vi "Main.vi"(5 "Instructions":bool, 7 "Stop":T2, 8 "Path to saved file":path, 9 "Load Button":bool, 10 "Track Button":T1, 11 "Target Button":bool) -> (3 "String":string)   [LabVIEW 2018]
doc: "This VI displays the orientation of an Android smartphone."
uses:
  stop control.ctl
  track control 2.ctl
panel:
  out "y axis degrees":dbl(knob) caption="x axis degrees" scale=-180.0..180.0
  out "XY Graph":cluster{"X":dbl, "Y":dbl}[](graph)
  out "x axis degrees":dbl(knob) scale=-180.0..180.0
  out "In y axis":dbl
  out "In x axis":dbl
  in  "Instructions panel":enum32{"Page 1", "Page 2"}(tab)
  in  "DOT":bool=TRUE
  # "Orientation from targeted position"
  # "degrees"
  # "degrees"
  # "First make sure the mobile and the computer are in the same network!\n1) Open the app \"IMU+GPS-Stream\"\n2) Write the appropriate IP address of the machine running Labview\n3) Select \"UDP Stream\"\n4) Change panel to \"Toggle Sensors\" and select \"Orientation\" and \"Include User-Checked Sensor Data in Stream\"\n5) At the Preferences panel click \"Switch Stream\" and point the mobile to the screen\n6) After having the mobile face the screen, you can press the TARGET button to start seeing the orientation of your phone in accordance to the targeting you've made\n7) Alternatively:\n  - Press the TRACK button BEFORE pressing the TARGET button  to also enable the recording of the data.\n   - Press the LOAD button (after selecting an appropriate file) to load already existing data and view the recording"
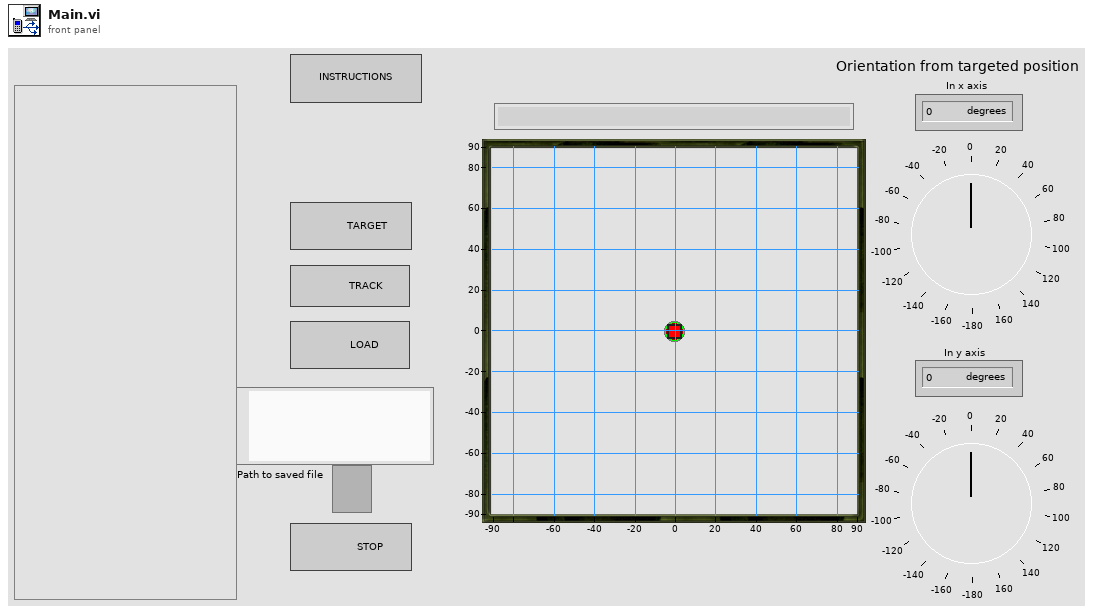
[diagram p1: front panel]
types:
  T1 = typedef "track control 2.ctl" = bool
  T2 = typedef "stop control.ctl" = bool
  T3 = enum16{"open", "replace", "create", "open or create", "replace or create", "replace or create with confirmation"}
  T4 = enum8{"Enabled", "Disabled", "Disabled and Grayed Out"}
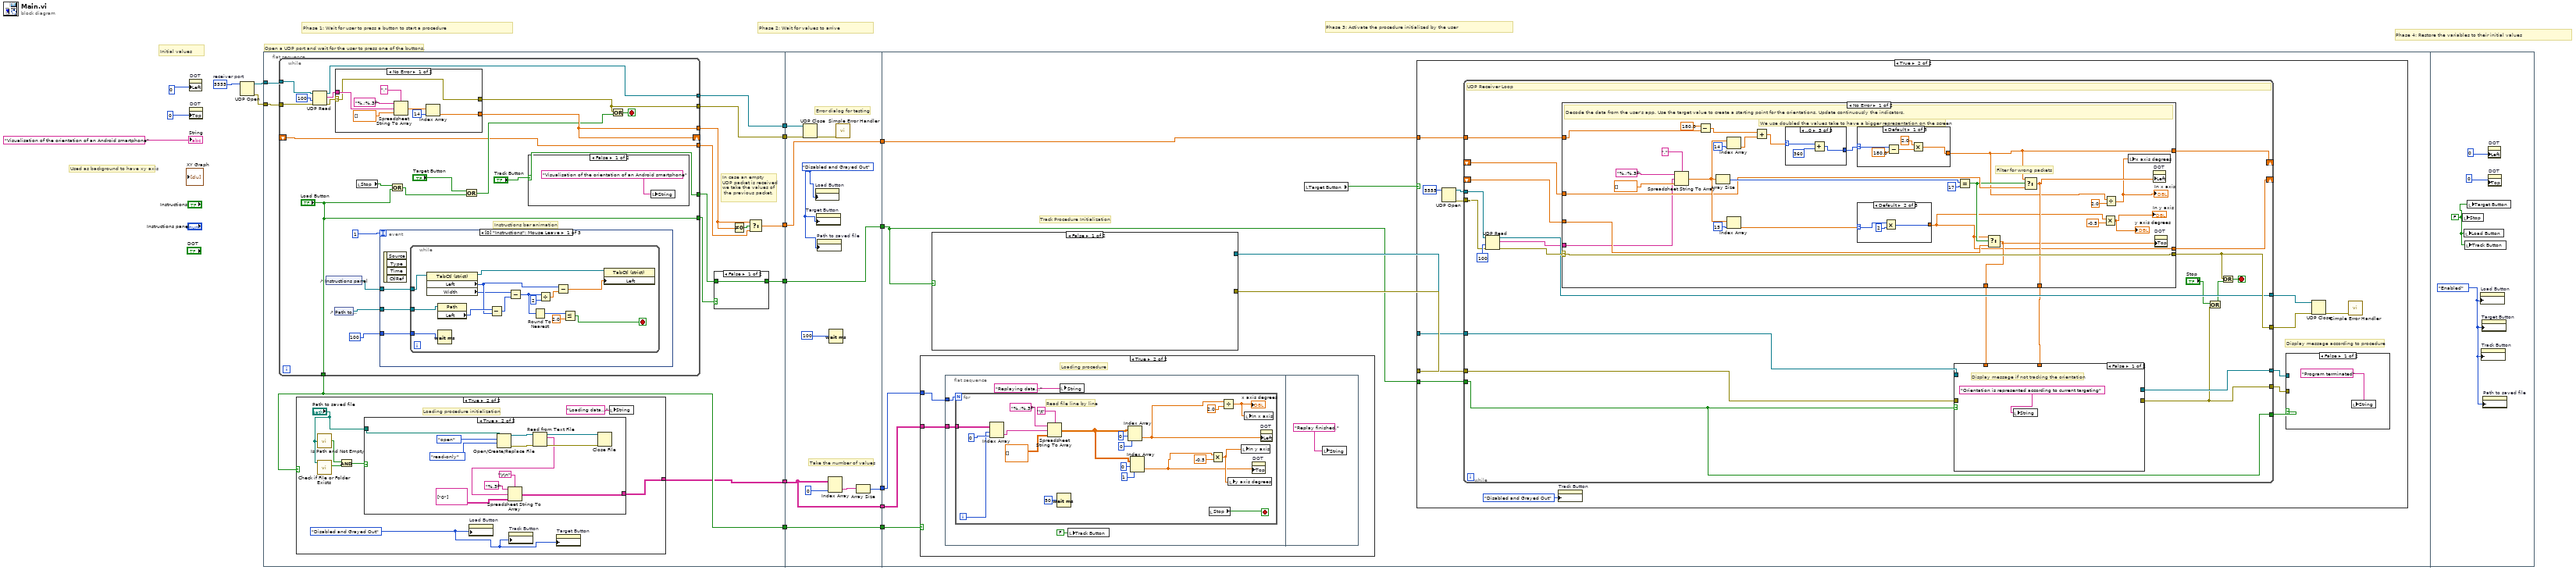
[diagram p0: block diagram]
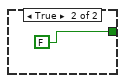
[diagram p2: hidden frame]
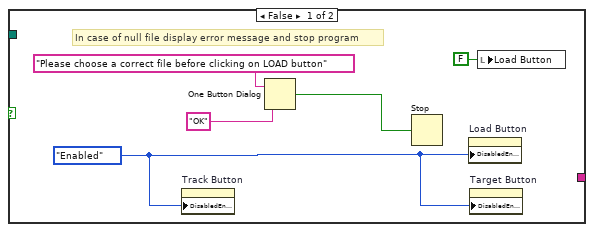
[diagram p4: hidden frame]
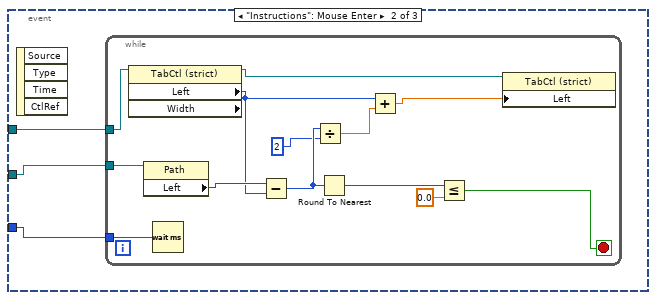
[diagram p5: hidden frame]
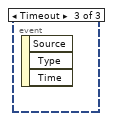
[diagram p6: hidden frame]
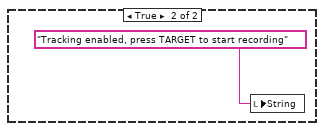
[diagram p7: hidden frame]
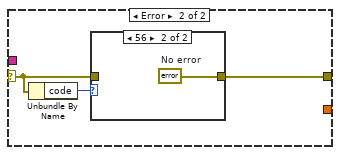
[diagram p8: hidden frame]
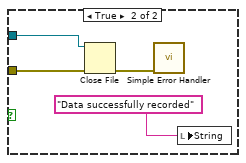
[diagram p11: hidden frame]
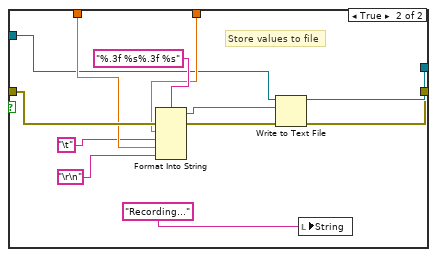
[diagram p12: hidden frame]
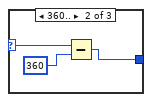
[diagram p14: hidden frame]
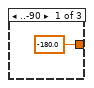
[diagram p15: hidden frame]
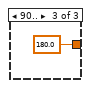
[diagram p16: hidden frame]
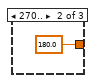
[diagram p17: hidden frame]
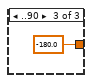
[diagram p18: hidden frame]
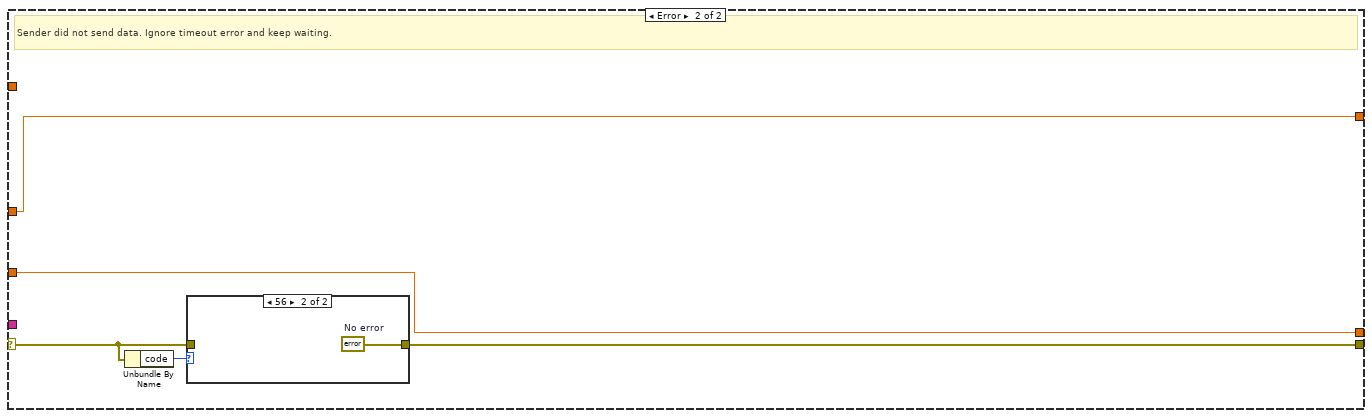
[diagram p19: hidden frame]
diagram:
  w17 = u16 5555  # receiver port
  # "Used as background to have xy axis"
  # "Phase 4: Restore the variables to their initial values"
  # "Phase 3: Activate the procedure initialized by the user"
  # "Phase 2: Wait for values to arrive"
  # "Phase 1: Wait for user to press a button to start a procedure"
  # "Open a UDP port and wait for the user to press one of the buttons."
  # "Initial values"
  n1 = property on="DOT" class="Bool (strict)"("Left"=0 ("Position:Left")) -> ()  [unwired: 2 in, 2 out]
  n2 = property on="DOT" class="Bool (strict)"("Top"=0 ("Position:Top")) -> ()  [unwired: 2 in, 2 out]
  n3 = UDP Open(11:w17) -> (port=w15:refnum<k16>, 0:w16:errorcluster)  [unwired: 4 in, 1 out]
  n4 = flat-sequence {
    tunnel: w15 -> [w28]
    tunnel: w16 -> [w27]
    tunnel: [w30] -> w14
    tunnel: [w29] -> w13
    tunnel: [w25] -> w12
    tunnel: [w22] -> w7
    tunnel: [w21] -> w5
    tunnel: [w18] -> w1
    tunnel: w14 -> [w135]
    tunnel: w13 -> [w136]
    tunnel: w12 -> [w134]
    tunnel: [w134] -> w11
    tunnel: [w133] -> w8
    tunnel: w7 -> [w133]
    tunnel: [w131] -> w6
    tunnel: w5 -> [w131]
    tunnel: [w129] -> w4
    tunnel: [w127] -> w2
    tunnel: w1 -> [w127]
    tunnel: w11 -> [w145]
    tunnel: w8 -> [w143]
    tunnel: w6 -> [w141]
    tunnel: w4 -> [w138]
    tunnel: w2 -> [w139]
    frame #0 {
      # "In case an empty\nUDP packet is received\nwe take the values of\n the previous packet."
      n5 = while {
        tunnel: w28 -> [w74]
        tunnel: [w72] -> w30
        tunnel: w27 -> [w75]
        tunnel: [w70] -> w29
        tunnel: [w69] -> w24
        shift-right: [w69] -> _
        shift-left: _ -> [w57]
        tunnel: [w57] -> w23
        tunnel: ["Load Button"] -> w22
        tunnel: ["Track Button"] -> w19
        tunnel: ["Load Button"] -> w20
        stop <- w62 stop-if-true
        # "Instructions bar animation"
        n6 = UDP Read(connection ID=w74, timeout ms (25000)=100, 8:w75) -> (data out=w73:string, error out=w71:errorcluster, 3:w72:refnum<k16>)  [unwired: 3 out]
        n7 = control-ref of="Instructions panel"() -> (w60:refnum<vi>)
        n8 = control-ref of="Path to saved file"() -> (w61:refnum<vi>)
        n9 = case shown="No Error" w71 {
          selector: w71 -> [w114 w122]
          tunnel: w73 -> [w116 _]
          tunnel: [w114 w121] -> w70
          tunnel: [w113 _] -> w69
          frame No Error {
            n10 = Spreadsheet String To Array(delimiter (Tab)=",", format string="%.;%.3f", spreadsheet string=w116, array type (2D Dbl)=dbl[] []) -> (array=w115:dbl[])
            n11 = Index Array(array=w115, index=14) -> (element=w113:dbl)
          }
          frame Error {
            n12 = Unbundle By Name(w122) -> ("code"=w123:i32)
            n13 = case shown="56" w123 {
              tunnel: w122 -> [w124 _]
              tunnel: [w124 w125] -> w121
              frame Default {
              }
              frame 56 {
                w125 = errorcluster {"status"=FALSE, "code"=0, "source"=""}  # No error
              }
            }
          }
        }
        n14 = local read "Stop"() -> (w66:T2)
        n15 = event shown="[0] \"Instructions\": Mouse Leave" {
          selector: _ -> [_ _ _]
          dyn-events: _ -> [_ _ _]
          timeout: 1 -> [_ _ _]
          tunnel: w61 -> [w79 w96 _]
          tunnel: w60 -> [w78 w95 _]
          tunnel: u32 100 ("Delay") -> [w77 w97 _]
          event "Instructions": Mouse Leave {
            n16 = event-data() -> ()  [unwired: 1 in, 4 out]
            n17 = while {
              tunnel: w79 -> [w91]
              tunnel: w78 -> [w90]
              tunnel: w77 -> [w89]
              stop <- w80 stop-if-true
              n18 = property on="Property Node" class="TabCtl (strict)"(reference=w90) -> (reference out=w92:refnum<vi>, "Left"=w93:i32, "Width"=w84:u32)  [unwired: 1 in, 1 out]
              n19 = property on="Property Node" class="Path"(reference=w91) -> ("Left"=w94:i32)  [unwired: 1 in, 2 out]
              n20 = Wait (ms)(milliseconds to wait=w89) -> ()  [unwired: 1 out]
              n21 = Subtract(x=w94, y=w93) -> (x-y=w87:i32)
              n22 = Subtract(x=w84, y=w87) -> (x-y=w88:u32)
              n23 = Round To Nearest(number=w88) -> (nearest integer value=w86:u32)
              n24 = Divide(x=w88, y=2) -> (x/y=w85:dbl)
              n25 = Subtract(x=w93, y=w85) -> (x-y=w81:dbl)
              n26 = Less Or Equal?(x=w86, y=2.0) -> (x <= y?=w80:bool)
              n27 = property on="Property Node" class="TabCtl (strict)"(reference=w92, "Left"=w81) -> ()  [unwired: 1 in, 2 out]
            }
          }
          event "Instructions": Mouse Enter {
            n28 = event-data() -> ()  [unwired: 1 in, 4 out]
            n29 = while {
              tunnel: w97 -> [w100]
              tunnel: w96 -> [w99]
              tunnel: w95 -> [w98]
              stop <- w101 stop-if-true
              n30 = property on="Property Node" class="TabCtl (strict)" props=["Left", "Width"](reference=w98) -> (reference out=w104:refnum<vi>, "Left"=w105:i32)  [unwired: 1 in, 2 out]
              n31 = property on="Property Node" class="Path"(reference=w99) -> ("Left"=w106:i32)  [unwired: 1 in, 2 out]
              n32 = Wait (ms)(milliseconds to wait=w100) -> ()  [unwired: 1 out]
              n33 = Subtract(x=w106, y=w105) -> (x-y=w107:i32)
              n34 = Divide(x=w107, y=2) -> (x/y=w109:dbl)
              n35 = Round To Nearest(number=w107) -> (nearest integer value=w108:i32)
              n36 = Add(x=w105, y=w109) -> (x+y=w110:dbl)
              n37 = Less Or Equal?(x=w108, y=0.0) -> (x <= y?=w101:bool)
              n38 = property on="Property Node" class="TabCtl (strict)"(reference=w104, "Left"=w110) -> ()  [unwired: 1 in, 2 out]
            }
          }
          event Timeout {
            n39 = event-data() -> ()  [unwired: 1 in, 3 out]
          }
        }
        n40 = Or(x=w66, y="Load Button") -> (x .or. y?=w65:T2)
        n41 = Or(x="Target Button", y=w65) -> (x .or. y?=w67:T2)
        n42 = case shown="False" "Track Button" {
          frame False {
            n43 = local write "String"("Visualisation of the orientation of an Android smartphone" ("String")) -> ()
          }
          frame True {
            n44 = local write "String"("Tracking enabled, press TARGET to start recording" ("String")) -> ()
          }
        }
        n45 = Or(x=w70, y=w67) -> (x .or. y?=w62:T2)
      }
      n46 = case shown="True" w22 {
        tunnel: [_ w39] -> w21
        frame False {
        }
        frame True {
          w33 = T4."Disabled and Grayed Out" ("Disabled")
          # "Loading procedure initialization"
          n47 = call <vilib>:"Is Path and Not Empty.vi"("path"="Path to saved file") -> ("Is Path and Not Empty?"=w36:bool)  [unwired: 4 in]
          n48 = call <vilib>:"Check if File or Folder Exists.vi"("path"="Path to saved file") -> ("file or folder exists?"=w37:bool)  [unwired: 8 in, 2 out]
          n49 = And(x=w36, y=w37) -> (x .and. y?=w35:bool)
          n50 = case shown="True" w35 {
            tunnel: [_ w46] -> w39
            tunnel: "Path to saved file" -> [_ w45]
            frame False {
              w41 = T4."Enabled" ("Disabled")
              # "In case of null file display error message and stop program"
              n51 = property on="Track Button" class="Bool (strict)"("DisabledEnum"=w41) -> ()  [unwired: 2 in, 2 out]
              n52 = One Button Dialog(message="Please choose a correct file before clicking on LOAD button", button name ("OK")="OK") -> (true=w42:bool)
              n53 = Stop(stop? (T)=w42) -> ()
              n54 = property on="Load Button" class="Bool (strict)"("DisabledEnum"=w41) -> ()  [unwired: 2 in, 2 out]
              n55 = property on="Target Button" class="Bool (strict)"("DisabledEnum"=w41) -> ()  [unwired: 2 in, 2 out]
              n56 = local write "Load Button"(FALSE ("Load Button")) -> ()
            }
            frame True {
              n57 = Open/Create/Replace File(file path (use dialog)=w45, operation (0:open)=T3."open", access (0:read/write)=enum16{"read/write", "read-only", "write-only"}."read-only") -> (refnum out=w51:refnum<file>, error out=w52:errorcluster)  [unwired: 3 in, 1 out]
              n58 = Read from Text File(file (use dialog)=w51, error in=w52) -> (refnum out=w56:refnum<file>, text=w50:string, error out=w55:errorcluster)  [unwired: 2 in, 1 out]
              n59 = Spreadsheet String To Array(delimiter (Tab)="\r\n", format string="%.3f", spreadsheet string=w50, array type (2D Dbl)=string[][] [["0"]]) -> (array=w46:string[][])
              n60 = Close File(refnum=w56, error in=w55) -> ()  [unwired: 2 out]
            }
          }
          n61 = property on="Load Button" class="Bool (strict)"("DisabledEnum"=w33) -> ()  [unwired: 2 in, 2 out]
          n62 = property on="Track Button" class="Bool (strict)"("DisabledEnum"=w33) -> ()  [unwired: 2 in, 2 out]
          n63 = property on="Target Button" class="Bool (strict)"("DisabledEnum"=w33) -> ()  [unwired: 2 in, 2 out]
          n64 = local write "String"("Loading data..." ("String")) -> ()
        }
      }
      n65 = case shown="False" w20 {
        tunnel: w19 -> [w31 _]
        tunnel: [w31 FALSE ("Track Button")] -> w18
        frame False {
        }
        frame True {
        }
      }
      n66 = Not Equal To 0?(x=w24) -> (x != 0?=w26:bool)
      n67 = Select(t=w24, s=w26, f=w23) -> (s? t:f=w25:dbl)
    }
    frame #1 {
      w126 = T4."Disabled and Grayed Out" ("Disabled")
      # "Error dialog for testing"
      # "Take the number of values"
      n68 = UDP Close(connection ID=w135, 8:w136) -> (error out=w128:errorcluster)  [unwired: 1 out]
      n69 = property on="Load Button" class="Bool (strict)"("DisabledEnum"=w126) -> ()  [unwired: 2 in, 2 out]
      n70 = property on="Target Button" class="Bool (strict)"("DisabledEnum"=w126) -> ()  [unwired: 2 in, 2 out]
      n71 = property on="Path to saved file" class="Path"("DisabledEnum"=w126) -> ()  [unwired: 2 in, 2 out]
      n72 = Index Array "Index Array"(array=w131, index (col)=0 ("index (row)")) -> (element=w130:string[])  [unwired: 1 in]
      n73 = Wait (ms)(milliseconds to wait=u32 100) -> ()  [unwired: 1 out]
      n74 = call <vilib>:"Simple Error Handler.vi"("error in (no error)"=w128) -> ()  [unwired: 1 in, 8 out]
      n75 = Array Size(array=w130) -> (size(s)=w129:i32)
    }
    frame #2 {
      # "Track Procedure Initialization"
      n76 = case shown="True" w143 {
        tunnel: w141 -> [_ w255]
        tunnel: w138 -> [_ w254]
        frame False {
        }
        frame True {
          # "Loading procedure"
          n77 = flat-sequence {
            tunnel: w255 -> [w259]
            tunnel: w254 -> [w258]
            frame #0 {
              n78 = for {
                N: w258 -> [_]
                tunnel: w259 -> [w279]
                i -> [w273]
                stop <- w266 stop-if-true
                # "Read file line by line"
                n79 = Index Array(array=w279, index (row)=w273, index (col)=0 ("index (row)")) -> (element=w278:string)
                n80 = Spreadsheet String To Array(delimiter (Tab)="\t", format string="%.;%.3f", spreadsheet string=w278, array type (2D Dbl)=dbl[][] []) -> (array=w268:dbl[][])
                n81 = Wait (ms)(milliseconds to wait=u32 50) -> ()  [unwired: 1 out]
                n82 = Index Array(array=w268, index (row)=0, index (col)=0 ("disabled index (col)")) -> (element=w261:dbl)
                n83 = Index Array(array=w268, index (row)=0, index (col)=1 ("disabled index (col)")) -> (element=w260:dbl)
                n84 = local read "Stop"() -> (w266:T2)
                n85 = Multiply(x=w260, y=-0.5) -> (x*y=w262:dbl)
                n86 = Divide(x=w261, y=2.0) -> (x/y=w263:dbl)
                "x axis degrees" <- w263
                n87 = local write "y axis degrees"(w262) -> ()
                n88 = local write "In y axis"(w262) -> ()
                n89 = local write "In x axis"(w263) -> ()
                n90 = property on="DOT" class="Bool (strict)"("Top"=w260) -> ()  [unwired: 2 in, 2 out]
                n91 = property on="DOT" class="Bool (strict)"("Left"=w261) -> ()  [unwired: 2 in, 2 out]
              }
              n92 = local write "String"("Replaying data..." ("String")) -> ()
              n93 = local write "Track Button"(FALSE ("Track Button")) -> ()
            }
            frame #1 {
              n94 = local write "String"("Replay finished." ("String")) -> ()
            }
          }
        }
      }
      n95 = case shown="False" w139 {
        tunnel: [_ w289] -> w144
        tunnel: [_ w282] -> w142
        frame False {
        }
        frame True {
          n96 = Format Date/Time String(time format string (%c)="%d%m%y_%H%M%S") -> (date/time string=w286:string)  [unwired: 2 in]
          n97 = Concatenate Strings "Concatenate Strings"("Measurements_" ("string"), w286, ".txt" ("string")) -> (w284:string)
          n98 = Build Path(base path=path "C:/Program Files/National Instruments/LabVIEW 2018/examples/My examples/My project/Saved Files", name or relative path=w284) -> (appended path=w283:path)
          n99 = Open/Create/Replace File(file path (use dialog)=w283, operation (0:open)=T3."replace or create") -> (refnum out=w282:refnum<file>, error out=w289:errorcluster)  [unwired: 4 in, 1 out]
        }
      }
      n100 = local read "Target Button"() -> (w140:bool)
      n101 = case shown="True" w140 {
        tunnel: w145 -> [_ w156]
        tunnel: w144 -> [_ w155]
        tunnel: w139 -> [_ w149]
        tunnel: w142 -> [_ w147]
        frame False {
        }
        frame True {
          # "Display message according to procedure"
          n102 = UDP Open(11:u16 5555) -> (port=w158:refnum<k16>, 0:w157:errorcluster)  [unwired: 4 in, 1 out]
          n103 = while {
            tunnel: [w185] -> w153
            shift-right: [w184] -> _
            shift-left: _ -> [w183]
            shift-right: [w182] -> _
            shift-left: _ -> [w181]
            tunnel: w158 -> [w179]
            tunnel: w157 -> [w178]
            tunnel: [w176] -> w152
            tunnel: w156 -> [w174]
            tunnel: w155 -> [w173]
            tunnel: [w171] -> w151
            tunnel: [w172] -> w150
            tunnel: w149 -> [w168]
            tunnel: [w168] -> w148
            tunnel: w147 -> [w167]
            stop <- w186 stop-if-true
            # "UDP Receiver Loop"
            n104 = UDP Read(connection ID=w179, timeout ms (25000)=100, 8:w178) -> (data out=w175:string, error out=w177:errorcluster, 3:w176:refnum<k16>)  [unwired: 3 out]
            n105 = case shown="No Error" w177 {
              selector: w177 -> [w227 w250]
              tunnel: [w227 w249] -> w185
              tunnel: [w201 w248] -> w184
              tunnel: w183 -> [w218 w248]
              tunnel: [w200 w247] -> w182
              tunnel: w181 -> [w216 w247]
              tunnel: w175 -> [w215 _]
              tunnel: w174 -> [w212 _]
              tunnel: [w207 _] -> w166
              tunnel: [w206 _] -> w165
              frame No Error {
                # "Filter for wrong packets"
                # "We use doubled the values take to have a bigger representation on the screen"
                # "Decode the data from the user's app. Use the target value to create a starting point for the orientations. Update continuously the indicators."
                n106 = Spreadsheet String To Array(delimiter (Tab)=",", format string="%.;%.3f", spreadsheet string=w215, array type (2D Dbl)=dbl[] []) -> (array=w219:dbl[])
                n107 = Subtract(x=180.0, y=w212) -> (x-y=w210:dbl)
                n108 = Array Size(array=w219) -> (size(s)=w221:i32)
                n109 = Index Array(array=w219, index=14) -> (element=w214:dbl)
                n110 = Index Array(array=w219, index=15) -> (element=w213:dbl)
                n111 = Add(x=w210, y=w214) -> (x+y=w209:dbl)
                n112 = case shown="..0" w209 {
                  selector: w209 -> [w228 w231 w234]
                  tunnel: [w228 w229 w232] -> w208
                  frame Default {
                  }
                  frame 360.. {
                    n113 = Subtract(x=w231, y=360) -> (x-y=w229:i32)
                  }
                  frame ..0 {
                    n114 = Add(x=w234, y=360) -> (x+y=w232:i32)
                  }
                }
                n115 = case shown="Default" w208 {
                  selector: w208 -> [w243 _ _]
                  tunnel: [w240 180.0 ("x") -180.0 ("x")] -> w201
                  frame Default {
                    n116 = Subtract(x=w243, y=180.0) -> (x-y=w241:dbl)
                    n117 = Multiply(x=2.0, y=w241) -> (x*y=w240:dbl)
                  }
                  frame 270.. {
                  }
                  frame ..90 {
                  }
                }
                n118 = case shown="Default" w213 {
                  selector: w213 -> [_ w238 _]
                  tunnel: [-180.0 ("x") w236 180.0 ("x")] -> w200
                  frame ..-90 {
                  }
                  frame Default {
                    n119 = Multiply(x=w238, y=2) -> (x*y=w236:i32)
                  }
                  frame 90.. {
                  }
                }
                n120 = Equal?(x=w221, y=17) -> (x = y?=w217:bool)
                n121 = Select(t=w200, s=w217, f=w216) -> (s? t:f=w206:dbl)
                n122 = Select(t=w201, s=w217, f=w218) -> (s? t:f=w207:dbl)
                n123 = Multiply(x=w200, y=-0.5) -> (x*y=→"In y axis" →"y axis degrees":dbl)
                n124 = Divide(x=w201, y=2.0) -> (x/y=w203:dbl)
                "In x axis" <- w203
                n125 = local write "x axis degrees"(w203) -> ()
                n126 = property on="DOT" class="Bool (strict)"("Left"=w207) -> ()  [unwired: 2 in, 2 out]
                n127 = property on="DOT" class="Bool (strict)"("Top"=w206) -> ()  [unwired: 2 in, 2 out]
              }
              frame Error {
                # "Sender did not send data. Ignore timeout error and keep waiting."
                n128 = Unbundle By Name(w250) -> ("code"=w251:i32)
                n129 = case shown="56" w251 {
                  tunnel: w250 -> [w252 _]
                  tunnel: [w252 w253] -> w249
                  frame Default {
                  }
                  frame 56 {
                    w253 = errorcluster {"status"=FALSE, "code"=0, "source"=""}  # No error
                  }
                }
              }
            }
            n130 = case shown="False" w168 {
              tunnel: w173 -> [_ w199]
              tunnel: [_ w197] -> w172
              tunnel: [_ w196] -> w171
              tunnel: w166 -> [_ w194]
              tunnel: w165 -> [_ w193]
              tunnel: w167 -> [_ w189]
              frame False {
                # "Display message if not tracking the orientation"
                n131 = local write "String"("Orientation is represented according to current targeting" ("String")) -> ()
              }
              frame True {
                # "Store values to file"
                n132 = Format Into String "Format Into String"(format string="%.3f %s%.3f %s", error in=w199, w194, "\t", w193, "\r\n") -> (resulting string=w190:string, error out=w198:errorcluster)  [unwired: 1 in]
                n133 = Write to Text File(file (use dialog)=w189, text=w190, error in=w198) -> (refnum out=w197:refnum<file>, error out=w196:errorcluster)  [unwired: 1 in, 1 out]
                n134 = local write "String"("Recording..." ("String")) -> ()
              }
            }
            n135 = Or(x="Stop", y=w171) -> (x .or. y?=w169:T2)
            n136 = Or(x=w185, y=w169) -> (x .or. y?=w186:T2)
          }
          n137 = property on="Track Button" class="Bool (strict)"("DisabledEnum"=T4."Disabled and Grayed Out" ("Disabled")) -> ()  [unwired: 2 in, 2 out]
          n138 = case shown="False" w148 {
            tunnel: w151 -> [_ w163]
            tunnel: w150 -> [_ w162]
            frame False {
              n139 = local write "String"("Program terminated" ("String")) -> ()
            }
            frame True {
              n140 = Close File(refnum=w162, error in=w163) -> (error out=w164:errorcluster)  [unwired: 1 out]
              n141 = call <vilib>:"Simple Error Handler.vi"("error in (no error)"=w164) -> ()  [unwired: 4 in, 5 out]
              n142 = local write "String"("Data successfully recorded" ("String")) -> ()
            }
          }
          n143 = UDP Close(connection ID=w152, 8:w153) -> (error out=w154:errorcluster)  [unwired: 1 out]
          n144 = call <vilib>:"Simple Error Handler.vi"("error in (no error)"=w154) -> ()  [unwired: 1 in, 8 out]
        }
      }
    }
    frame #3 {
      w293 = T4."Enabled" ("Disabled")
      w294 = FALSE ("Stop")
      n145 = local write "Stop"(w294) -> ()
      n146 = local write "Load Button"(w294) -> ()
      n147 = local write "Track Button"(w294) -> ()
      n148 = local write "Target Button"(w294) -> ()
      n149 = property on="Load Button" class="Bool (strict)"("DisabledEnum"=w293) -> ()  [unwired: 2 in, 2 out]
      n150 = property on="Track Button" class="Bool (strict)"("DisabledEnum"=w293) -> ()  [unwired: 2 in, 2 out]
      n151 = property on="Target Button" class="Bool (strict)"("DisabledEnum"=w293) -> ()  [unwired: 2 in, 2 out]
      n152 = property on="Path to saved file" class="Path"("DisabledEnum"=w293) -> ()  [unwired: 2 in, 2 out]
      n153 = property on="DOT" class="Bool (strict)"("Left"=0 ("Position:Left")) -> ()  [unwired: 2 in, 2 out]
      n154 = property on="DOT" class="Bool (strict)"("Top"=0 ("Position:Top")) -> ()  [unwired: 2 in, 2 out]
    }
  }
  "String" <- "Visualisation of the orientation of an Android smartphone" ("String")
